vi "Speed from Pulse Position (N Ch).vi"(4 "Offset":dbl, 6 "Scale":dbl, 7 "Speed From Pulse":T1, 8 "Min EU":dbl, 10 "Max Empty Blocks":dbl, 11 "speed position info":T2) -> (3 "Speed in EU":dbl format="%0.2f", 5 "Speed From Pulse":T1)   [LabVIEW 2018, in "Measurement Channels.lvlib" / "Tachometer.lvclass"]
uses:
  Tachometer.lvclass
  <vilib>/addons/Sound and Vibration/Order Analysis/Misc/OAT Position Info.ctl
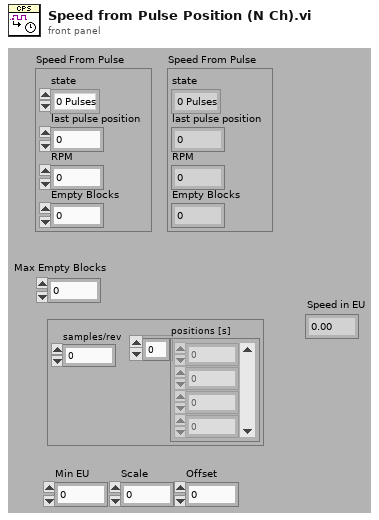
[diagram p1: front panel]
types:
  T1 = cluster{"state":enum16{"0 Pulses", "1 Pulse", "2+ Pulses"}, "last pulse position":dbl, "RPM":dbl, "Empty Blocks":i32}
  T2 = typedef "OAT Position Info.ctl" = cluster{"positions [s]":dbl[], "samples/rev":dbl}
  T3 = cluster{"state":enum16{"0 Pulses", "1 Pulse", "2+ Pulses"}, "last pulse position":dbl, "CPS":dbl, "Empty Blocks":i32}
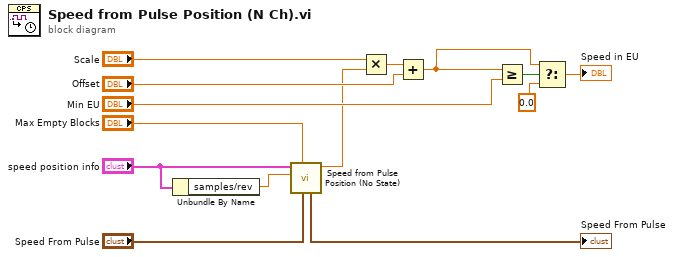
[diagram p0: block diagram]
diagram:
  n1 = Unbundle By Name("speed position info") -> ("samples/rev"=w8:dbl)
  n2 = call "Speed from Pulse Position (No State).vi"("state in"="Speed From Pulse", "Blocks/Pulse"="Max Empty Blocks", "pulse/revolution (1)"=w8, "speed position info"="speed position info") -> ("CPS"=w4:dbl, "state out"=→"Speed From Pulse":T3)  [unwired: 6 in]
  n3 = Multiply(x="Scale", y=w4) -> (x*y=w5:dbl)
  n4 = Add(x=w5, y="Offset") -> (x+y=w3:dbl)
  n5 = Greater Or Equal?(x=w3, y="Min EU") -> (x >= y?=w6:bool)
  n6 = Select(t=w3, s=w6, f=0.0 ("t")) -> (s? t:f=→"Speed in EU":dbl)
